vi "Generic command handler.vi"(8 "error in (no error)":errorcluster, 10 "Message in":refnum<class "GenericMessage.lvclass">, 11 "Tomo in":refnum<class "Tomo.lvclass">) -> (0 "error out":errorcluster, 2 "value":string, 3 "Tomo out":refnum<class "Tomo.lvclass">)   [LabVIEW 2012, in "Tomo.lvclass"]
doc: "The generic_command_handler processes the command 'generic'. Commands which are not part of the predefined list of commands fall under the 'generic' command for special activity."
uses:
  Tomo.lvclass
  <vilib>/Distrio/Murmex/GenericMessage/GenericMessage.lvclass
  <vilib>/Distrio/Murmex/Murmex/Murmex.lvclass
  <vilib>/Distrio/Murmex/StartMessage/StartMessage.lvclass
  file type.ctl
  notice type.ctl
  <vilib>/Distrio/Murmex/StopMessage/StopMessage.lvclass
  <vilib>/Distrio/Murmex/Message/Add or replace parameter.vi
  <vilib>/Distrio/Murmex/Message/Message.lvclass
panel:
  # "This method is called when the GENERIC\ntrigger is sent. \n\nOverride this method when your component needs to\nrespond to this trigger. \n\nCall parent for proper implementation"
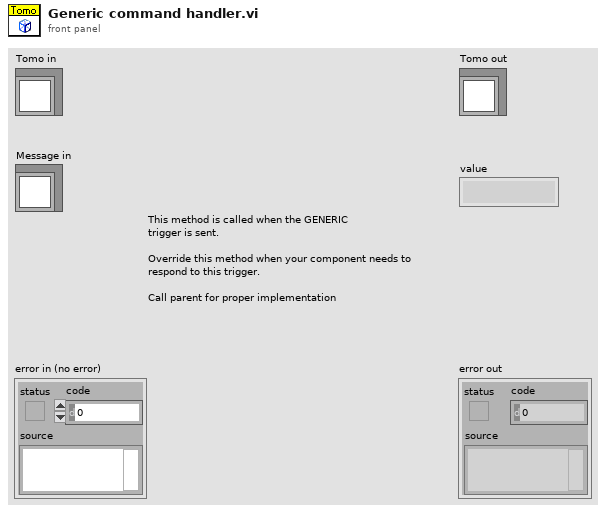
[diagram p1: front panel]
types:
  T1 = typedef "Tomo.lvclass/file type.ctl" = enum16{"Volume map", "Completed stacks"}
  T2 = typedef "Tomo.lvclass/notice type.ctl" = enum16{"Tomography stopped", "Tomography error", "Tomography finished", "Timing issue", "Critical timing issue"}
  T3 = typedef "Tomo.lvclass/volume map.ctl" = enum16{"Cubic volume", "Custom volume", "Self-generate volume"}
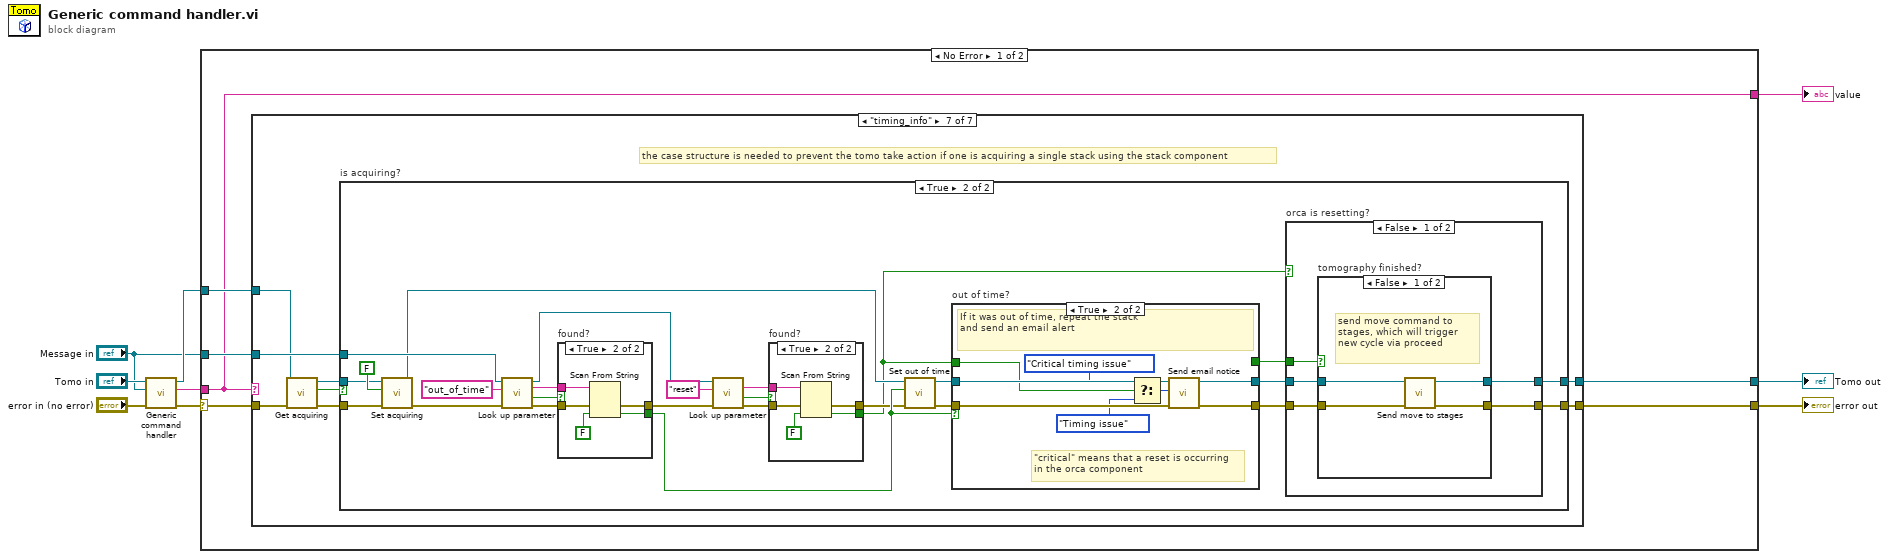
[diagram p0: block diagram]
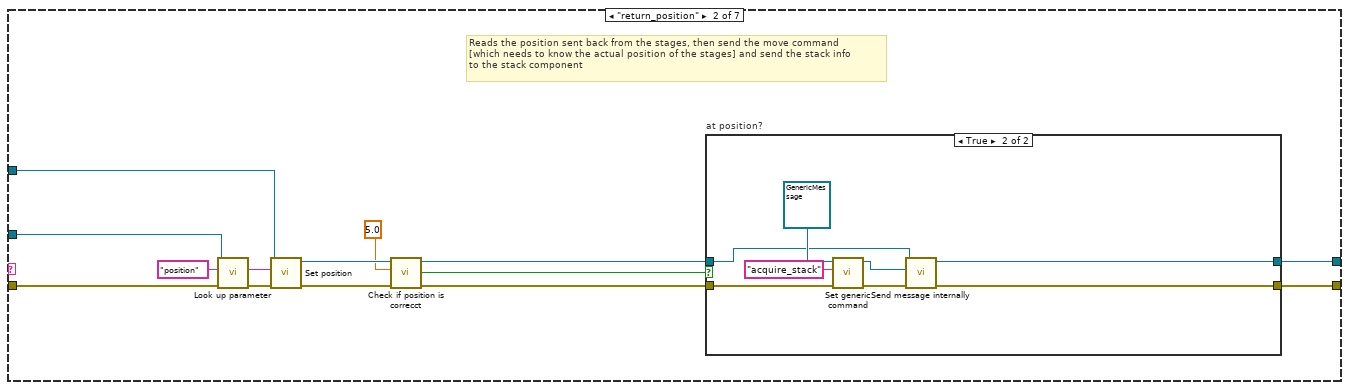
[diagram p3: hidden frame]
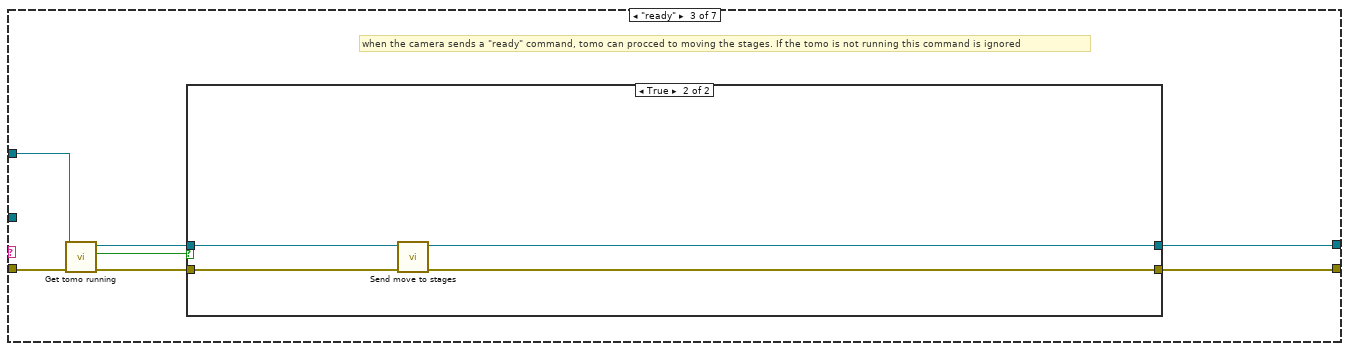
[diagram p5: hidden frame]
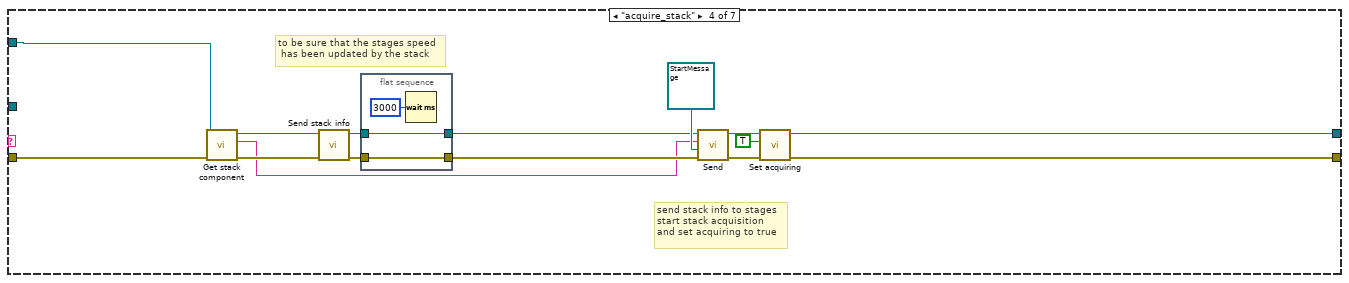
[diagram p7: hidden frame]
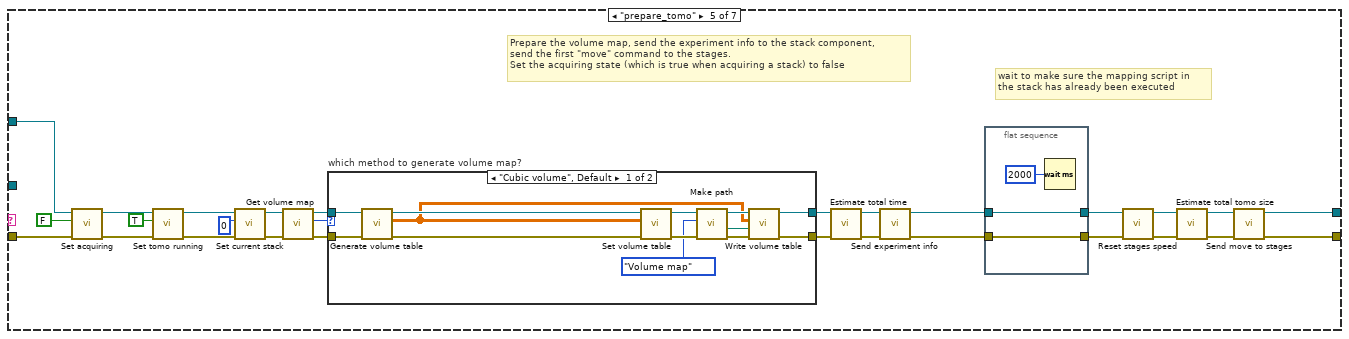
[diagram p8: hidden frame]
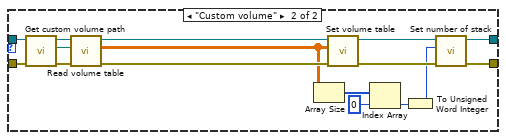
[diagram p9: hidden frame]
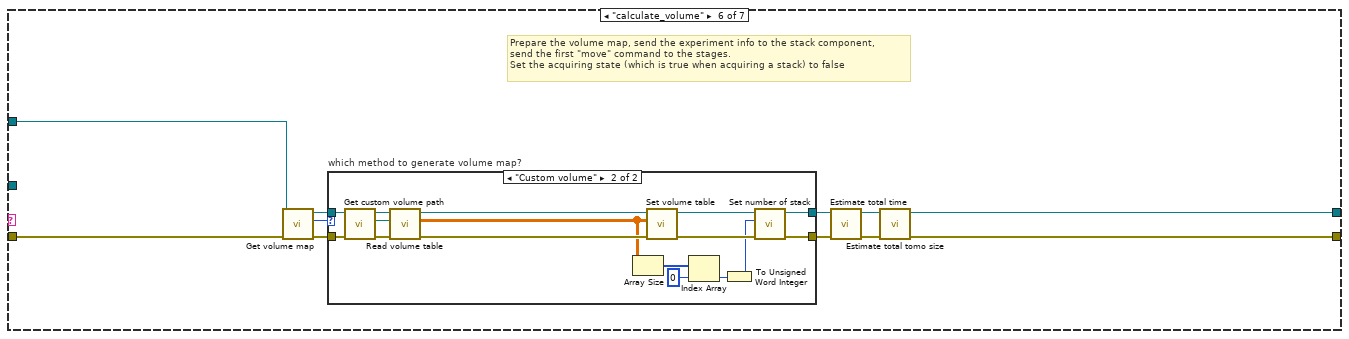
[diagram p10: hidden frame]
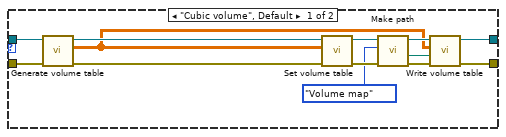
[diagram p11: hidden frame]
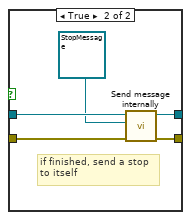
[diagram p13: hidden frame]
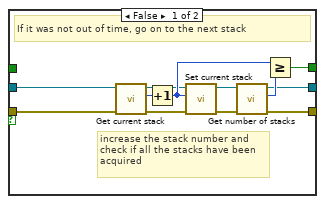
[diagram p16: hidden frame]
diagram:
  n1 = call-parent "Generic command handler.vi"("error in (no error)"="error in (no error)", "Message in"="Message in", "Murmex in"="Tomo in") -> ("error out"=w7:errorcluster, "value"=w6:string, "Murmex out"=w5:refnum<class "Tomo.lvclass">)  [unwired: 6 in]
  n2 = case shown="No Error" w7 {
    selector: w7 -> [w15 w257]
    tunnel: w6 -> [w11 w259]
    tunnel: w5 -> [w14 w258]
    tunnel: "Message in" -> [w13 _]
    tunnel: [w12 w258] -> w3
    tunnel: [w11 w259] -> w2
    tunnel: [w10 w257] -> w1
    frame No Error {
      n3 = case shown="\"timing_info\"" w11 {
        tunnel: w15 -> [w17 w31 w48 w61 w93 w139 w177]
        tunnel: w14 -> [w16 w30 w47 w59 w91 w138 w175]
        tunnel: w13 -> [_ w29 _ _ _ _ w180]
        tunnel: [w17 w19 w44 w56 w86 w135 w178] -> w10
        tunnel: [w16 w18 w42 w55 w85 w133 w179] -> w12
        frame Default {
        }
        frame "return_position" {
          # "Reads the position sent back from the stages, then send the move command\n[which needs to know the actual position of the stages] and send the stack info\nto the stack component"
          n4 = call <vilib>:"Look up parameter.vi"("error in (no error)"=w31, "name"="position", "Message in"=w29) -> ("error out"=w27:errorcluster, "key"=w26:string)  [unwired: 5 in, 2 out]
          n5 = call-dynamic "Set position.vi"("error in (no error)"=w27, "XML in"=w26, "Tomo in"=w30) -> ("error out"=w25:errorcluster, "Tomo out"=w24:refnum<class "Tomo.lvclass">)  [unwired: 7 in]
          n6 = call-dynamic "Check if position is correcct.vi"("error in (no error)"=w25, "Tolerance (um)"=5.0 ("Tolerance"), "Tomo in"=w24) -> ("error out"=w21:errorcluster, "correct?"=w22:bool, "Tomo out"=w20:refnum<class "Tomo.lvclass">)  [unwired: 6 in]
          n7 = case "at position?" shown="True" w22 {
            tunnel: w21 -> [w33 w40]
            tunnel: w20 -> [w32 w36]
            tunnel: [w33 w35] -> w19
            tunnel: [w32 w34] -> w18
            frame False {
            }
            frame True {
              n8 = call <vilib>:"Set generic command.vi"("error in (no error)"=w40, "generic command"="acquire_stack", "GenericMessage in"=refnum<class "GenericMessage.lvclass"> refnum ("Distrio Murmex 1.2:GenericMessage")) -> ("error out"=w41:errorcluster, "GenericMessage out"=w37:refnum<class "GenericMessage.lvclass">)  [unwired: 7 in]
              n9 = call <vilib>:"Send message internally.vi"("error in (no error)"=w41, "Message"=w37, "Murmex in"=w36) -> ("error out"=w35:errorcluster, "Murmex out"=w34:refnum<class "Tomo.lvclass">)  [unwired: 7 in]
            }
          }
        }
        frame "ready" {
          # "when the camera sends a \"ready\" command, tomo can procced to moving the stages. If the tomo is not running this command is ignored"
          n10 = call-dynamic "Get tomo running.vi"("error in (no error)"=w48, "Tomo in"=w47) -> ("error out"=w45:errorcluster, "tomo running?"=w46:bool, "Tomo out"=w43:refnum<class "Tomo.lvclass">)  [unwired: 7 in]
          n11 = case shown="True" w46 {
            tunnel: w45 -> [w49 w54]
            tunnel: [w49 w53] -> w44
            tunnel: w43 -> [w50 w52]
            tunnel: [w50 w51] -> w42
            frame False {
            }
            frame True {
              n12 = call-dynamic "Send move to stages.vi"("error in (no error)"=w54, "Tomo in"=w52) -> ("error out"=w53:errorcluster, "Tomo out"=w51:refnum<class "Tomo.lvclass">)  [unwired: 8 in]
            }
          }
        }
        frame "acquire_stack" {
          # "to be sure that the stages speed\n has been updated by the stack"
          # "send stack info to stages\nstart stack acquisition\nand set acquiring to true"
          n13 = call-dynamic "Get stack component.vi"("error in (no error)"=w61, "Tomo in"=w59) -> ("error out"=w60:errorcluster, "stack component"=w57:string, "Tomo out"=w58:refnum<class "Tomo.lvclass">)  [unwired: 7 in]
          n14 = call-dynamic "Send stack info.vi"("error in (no error)"=w60, "Tomo in"=w58) -> ("error out"=w62:errorcluster, "Tomo out"=w64:refnum<class "Tomo.lvclass">)  [unwired: 8 in]
          n15 = flat-sequence {
            tunnel: [w72] -> w65
            tunnel: w64 -> [w72]
            tunnel: [w71] -> w63
            tunnel: w62 -> [w71]
            frame #0 {
              n16 = Wait (ms)(milliseconds to wait=u32 3000) -> ()  [unwired: 1 out]
            }
          }
          n17 = call <vilib>:"Send.vi"("error in (no error)"=w63, "Message"=refnum<class "StartMessage.lvclass"> refnum ("Message in"), "recipient"=w57, "Murmex in"=w65) -> ("error out"=w69:errorcluster, "Murmex out"=w68:refnum<class "Tomo.lvclass">)  [unwired: 6 in]
          n18 = call-dynamic "Set acquiring.vi"("error in (no error)"=w69, "is acquiring?"=TRUE, "Tomo in"=w68) -> ("error out"=w56:errorcluster, "Tomo out"=w55:refnum<class "Tomo.lvclass">)  [unwired: 7 in]
        }
        frame "prepare_tomo" {
          # "wait to make sure the mapping script in \nthe stack has already been executed"
          # "Prepare the volume map, send the experiment info to the stack component,\nsend the first \"move\" command to the stages.\nSet the acquiring state (which is true when acquiring a stack) to false"
          n19 = call-dynamic "Set acquiring.vi"("error in (no error)"=w93, "is acquiring?"=FALSE, "Tomo in"=w91) -> ("error out"=w92:errorcluster, "Tomo out"=w82:refnum<class "Tomo.lvclass">)  [unwired: 7 in]
          n20 = call-dynamic "Set tomo running.vi"("error in (no error)"=w92, "tomo running?"=TRUE, "Tomo in"=w82) -> ("error out"=w77:errorcluster, "Tomo out"=w78:refnum<class "Tomo.lvclass">)  [unwired: 7 in]
          n21 = call-dynamic "Set current stack.vi"("error in (no error)"=w77, "Current stack"=u16 0, "Tomo in"=w78) -> ("error out"=w96:errorcluster, "Tomo out"=w97:refnum<class "Tomo.lvclass">)  [unwired: 7 in]
          n22 = call-dynamic "Get volume map.vi"("error in (no error)"=w96, "Tomo in"=w97) -> ("error out"=w99:errorcluster, "Volume map"=w100:T3, "Tomo out"=w98:refnum<class "Tomo.lvclass">)  [unwired: 7 in]
          n23 = case "which method to generate volume map?" shown="\"Cubic volume\", Default" w100 {
            tunnel: w99 -> [w115 w130]
            tunnel: w98 -> [w116 w128]
            tunnel: [w105 w122] -> w88
            tunnel: [w104 w124] -> w94
            frame "Cubic volume", Default {
              n24 = call-dynamic "Generate volume table.vi"("error in (no error)"=w115, "Tomo in"=w116) -> ("error out"=w113:errorcluster, "Volume table"=w106:dbl[][], "Tomo out"=w114:refnum<class "Tomo.lvclass">)  [unwired: 7 in]
              n25 = call-dynamic "Set volume table.vi"("error in (no error)"=w113, "Volume map in"=w106, "Tomo in"=w114) -> ("error out"=w111:errorcluster, "Tomo out"=w112:refnum<class "Tomo.lvclass">)  [unwired: 7 in]
              n26 = call-dynamic "Make path.vi"("error in (no error)"=w111, "File type"=file_type."Volume map", "Tomo in"=w112) -> ("error out"=w108:errorcluster, "path"=w107:path, "Tomo out"=w109:refnum<class "Tomo.lvclass">)  [unwired: 6 in]
              n27 = call-dynamic "Write volume table.vi"("error in (no error)"=w108, "File name"=w107, "Volume map"=w106, "Tomo in"=w109) -> ("error out"=w104:errorcluster, "Tomo out"=w105:refnum<class "Tomo.lvclass">)  [unwired: 6 in]
            }
            frame "Custom volume" {
              n28 = call-dynamic "Get custom volume path.vi"("error in (no error)"=w130, "Tomo in"=w128) -> ("error out"=w129:errorcluster, "Custom volume path"=w126:path, "Tomo out"=w127:refnum<class "Tomo.lvclass">)  [unwired: 7 in]
              n29 = call-dynamic "Read volume table.vi"("error in (no error)"=w129, "File path"=w126, "Tomo in"=w127) -> ("error out"=w131:errorcluster, "System Array"=w118:dbl[][], "Tomo out"=w132:refnum<class "Tomo.lvclass">)  [unwired: 6 in]
              n30 = Array Size(array=w118) -> (size(s)=w121:i32[])
              n31 = call-dynamic "Set volume table.vi"("error in (no error)"=w131, "Volume map in"=w118, "Tomo in"=w132) -> ("error out"=w125:errorcluster, "Tomo out"=w123:refnum<class "Tomo.lvclass">)  [unwired: 7 in]
              n32 = Index Array(array=w121, index=0) -> (element=w119:i32)
              n33 = To Unsigned Word Integer(number=w119) -> (unsigned 16bit integer=w117:u16)
              n34 = call-dynamic "Set number of stack.vi"("error in (no error)"=w125, "Number of stacks"=w117, "Tomo in"=w123) -> ("error out"=w124:errorcluster, "Tomo out"=w122:refnum<class "Tomo.lvclass">)  [unwired: 7 in]
            }
          }
          n35 = call-dynamic "Estimate total time.vi"("error in (no error)"=w94, "Tomo in"=w88) -> ("error out"=w89:errorcluster, "Tomo out"=w87:refnum<class "Tomo.lvclass">)  [unwired: 8 in]
          n36 = call-dynamic "Send experiment info.vi"("error in (no error)"=w89, "Tomo in"=w87) -> ("error out"=w73:errorcluster, "Tomo out"=w75:refnum<class "Tomo.lvclass">)  [unwired: 8 in]
          n37 = flat-sequence {
            tunnel: [w103] -> w76
            tunnel: w75 -> [w103]
            tunnel: [w102] -> w74
            tunnel: w73 -> [w102]
            frame #0 {
              n38 = Wait (ms)(milliseconds to wait=u32 2000) -> ()  [unwired: 1 out]
            }
          }
          n39 = call-dynamic "Reset stages speed.vi"("error in (no error)"=w74, "Tomo in"=w76) -> ("error out"=w80:errorcluster, "Tomo out"=w79:refnum<class "Tomo.lvclass">)  [unwired: 8 in]
          n40 = call "Estimate total tomo size.vi"("error in (no error)"=w80, "Tomo in"=w79) -> ("error out"=w84:errorcluster, "Tomo out"=w83:refnum<class "Tomo.lvclass">)  [unwired: 7 in, 1 out]
          n41 = call-dynamic "Send move to stages.vi"("error in (no error)"=w84, "Tomo in"=w83) -> ("error out"=w86:errorcluster, "Tomo out"=w85:refnum<class "Tomo.lvclass">)  [unwired: 8 in]
        }
        frame "calculate_volume" {
          # "Prepare the volume map, send the experiment info to the stack component,\nsend the first \"move\" command to the stages.\nSet the acquiring state (which is true when acquiring a stack) to false"
          n42 = call-dynamic "Get volume map.vi"("error in (no error)"=w139, "Tomo in"=w138) -> ("error out"=w142:errorcluster, "Volume map"=w143:T3, "Tomo out"=w141:refnum<class "Tomo.lvclass">)  [unwired: 7 in]
          n43 = case "which method to generate volume map?" shown="\"Custom volume\"" w143 {
            tunnel: w142 -> [w155 w170]
            tunnel: w141 -> [w156 w168]
            tunnel: [w145 w162] -> w137
            tunnel: [w144 w164] -> w140
            frame "Cubic volume", Default {
              n44 = call-dynamic "Generate volume table.vi"("error in (no error)"=w155, "Tomo in"=w156) -> ("error out"=w153:errorcluster, "Volume table"=w146:dbl[][], "Tomo out"=w154:refnum<class "Tomo.lvclass">)  [unwired: 7 in]
              n45 = call-dynamic "Set volume table.vi"("error in (no error)"=w153, "Volume map in"=w146, "Tomo in"=w154) -> ("error out"=w151:errorcluster, "Tomo out"=w152:refnum<class "Tomo.lvclass">)  [unwired: 7 in]
              n46 = call-dynamic "Make path.vi"("error in (no error)"=w151, "File type"=file_type."Volume map", "Tomo in"=w152) -> ("error out"=w148:errorcluster, "path"=w147:path, "Tomo out"=w149:refnum<class "Tomo.lvclass">)  [unwired: 6 in]
              n47 = call-dynamic "Write volume table.vi"("error in (no error)"=w148, "File name"=w147, "Volume map"=w146, "Tomo in"=w149) -> ("error out"=w144:errorcluster, "Tomo out"=w145:refnum<class "Tomo.lvclass">)  [unwired: 6 in]
            }
            frame "Custom volume" {
              n48 = call-dynamic "Get custom volume path.vi"("error in (no error)"=w170, "Tomo in"=w168) -> ("error out"=w169:errorcluster, "Custom volume path"=w166:path, "Tomo out"=w167:refnum<class "Tomo.lvclass">)  [unwired: 7 in]
              n49 = call-dynamic "Read volume table.vi"("error in (no error)"=w169, "File path"=w166, "Tomo in"=w167) -> ("error out"=w171:errorcluster, "System Array"=w158:dbl[][], "Tomo out"=w172:refnum<class "Tomo.lvclass">)  [unwired: 6 in]
              n50 = Array Size(array=w158) -> (size(s)=w161:i32[])
              n51 = call-dynamic "Set volume table.vi"("error in (no error)"=w171, "Volume map in"=w158, "Tomo in"=w172) -> ("error out"=w165:errorcluster, "Tomo out"=w163:refnum<class "Tomo.lvclass">)  [unwired: 7 in]
              n52 = Index Array(array=w161, index=0) -> (element=w159:i32)
              n53 = To Unsigned Word Integer(number=w159) -> (unsigned 16bit integer=w157:u16)
              n54 = call-dynamic "Set number of stack.vi"("error in (no error)"=w165, "Number of stacks"=w157, "Tomo in"=w163) -> ("error out"=w164:errorcluster, "Tomo out"=w162:refnum<class "Tomo.lvclass">)  [unwired: 7 in]
            }
          }
          n55 = call-dynamic "Estimate total time.vi"("error in (no error)"=w140, "Tomo in"=w137) -> ("error out"=w136:errorcluster, "Tomo out"=w134:refnum<class "Tomo.lvclass">)  [unwired: 8 in]
          n56 = call "Estimate total tomo size.vi"("error in (no error)"=w136, "Tomo in"=w134) -> ("error out"=w135:errorcluster, "Tomo out"=w133:refnum<class "Tomo.lvclass">)  [unwired: 7 in, 1 out]
        }
        frame "timing_info" {
          # "the case structure is needed to prevent the tomo take action if one is acquiring a single stack using the stack component"
          n57 = call-dynamic "Get acquiring.vi"("error in (no error)"=w177, "Tomo in"=w175) -> ("error out"=w176:errorcluster, "is acquiring?"=w173:bool, "Tomo out"=w174:refnum<class "Tomo.lvclass">)  [unwired: 7 in]
          n58 = case "is acquiring?" shown="True" w173 {
            tunnel: w180 -> [_ w208]
            tunnel: [w182 w201] -> w179
            tunnel: [w181 w200] -> w178
            tunnel: w176 -> [w181 w197]
            tunnel: w174 -> [w182 w195]
            frame False {
            }
            frame True {
              n59 = call-dynamic "Set acquiring.vi"("error in (no error)"=w197, "is acquiring?"=FALSE, "Tomo in"=w195) -> ("error out"=w196:errorcluster, "Tomo out"=w193:refnum<class "Tomo.lvclass">)  [unwired: 7 in]
              n60 = call <vilib>:"Look up parameter.vi"("error in (no error)"=w196, "name"="out_of_time", "Message in"=w208) -> ("error out"=w206:errorcluster, "found?"=w204:bool, "key"=w205:string, "Message out"=w185:refnum<class "GenericMessage.lvclass">)  [unwired: 5 in]
              n61 = case "found?" shown="True" w204 {
                tunnel: w206 -> [w251 w255]
                tunnel: w205 -> [_ w254]
                tunnel: [w251 w253] -> w184
                tunnel: [_ w252] -> w191
                frame False {
                }
                frame True {
                  n62 = Scan From String(input string=w254, error in=w255, default 1=FALSE) -> (error out=w253:errorcluster, output 1=w252:bool)  [unwired: 2 in, 2 out]
                }
              }
              n63 = call <vilib>:"Look up parameter.vi"("error in (no error)"=w184, "name"="reset", "Message in"=w185) -> ("error out"=w189:errorcluster, "found?"=w187:bool, "key"=w188:string)  [unwired: 5 in, 1 out]
              n64 = case "found?" shown="True" w187 {
                tunnel: w189 -> [w225 w229]
                tunnel: w188 -> [_ w228]
                tunnel: [w225 w227] -> w186
                tunnel: [_ w226] -> w183
                frame False {
                }
                frame True {
                  n65 = Scan From String(input string=w228, error in=w229, default 1=FALSE) -> (error out=w227:errorcluster, output 1=w226:bool)  [unwired: 2 in, 2 out]
                }
              }
              n66 = call-dynamic "Set out of time.vi"("error in (no error)"=w186, "out of time?"=w191, "Tomo in"=w193) -> ("error out"=w194:errorcluster, "Tomo out"=w192:refnum<class "Tomo.lvclass">)  [unwired: 7 in]
              n67 = case "out of time?" shown="True" w191 {
                tunnel: w194 -> [w235 w249]
                tunnel: w192 -> [w234 w250]
                tunnel: [w233 w248] -> w203
                tunnel: [w232 w247] -> w202
                tunnel: [w231 _] -> w199
                tunnel: w183 -> [_ w244]
                frame False {
                  # "increase the stack number and\ncheck if all the stacks have been\nacquired"
                  # "If it was not out of time, go on to the next stack"
                  n68 = call-dynamic "Get current stack.vi"("error in (no error)"=w235, "Tomo in"=w234) -> ("error out"=w237:errorcluster, "Current stack"=w238:u16, "Tomo out"=w236:refnum<class "Tomo.lvclass">)  [unwired: 7 in]
                  n69 = Increment(x=w238) -> (x+1=w242:u16)
                  n70 = call-dynamic "Set current stack.vi"("error in (no error)"=w237, "Current stack"=w242, "Tomo in"=w236) -> ("error out"=w239:errorcluster, "Tomo out"=w240:refnum<class "Tomo.lvclass">)  [unwired: 7 in]
                  n71 = call-dynamic "Get number of stacks.vi"("error in (no error)"=w239, "Tomo in"=w240) -> ("error out"=w233:errorcluster, "Number of stacks"=w241:u16, "Tomo out"=w232:refnum<class "Tomo.lvclass">)  [unwired: 7 in]
                  n72 = Greater Or Equal?(x=w242, y=w241) -> (x >= y?=w231:bool)
                }
                frame True {
                  # "\"critical\" means that a reset is occurring\nin the orca component"
                  # "If it was out of time, repeat the stack\nand send an email alert"
                  n73 = Select(t=notice_type."Critical timing issue" ("Notice type"), s=w244, f=notice_type."Timing issue" ("Notice type")) -> (s? t:f=w243:T2)
                  n74 = call-dynamic "Send email notice.vi"("error in (no error)"=w249, "Notice type"=w243, "Tomo in"=w250) -> ("error out"=w248:errorcluster, "Tomo out"=w247:refnum<class "Tomo.lvclass">)  [unwired: 7 in]
                }
              }
              n75 = case "orca is resetting?" shown="False" w183 {
                tunnel: w203 -> [w213 w224]
                tunnel: w202 -> [w212 w223]
                tunnel: [w211 w223] -> w201
                tunnel: [w210 w224] -> w200
                tunnel: w199 -> [w209 _]
                frame False {
                  n76 = case "tomography finished?" shown="False" w209 {
                    tunnel: w213 -> [w217 w222]
                    tunnel: w212 -> [w216 w219]
                    tunnel: [w215 w220] -> w211
                    tunnel: [w214 w221] -> w210
                    frame False {
                      # "send move command to stages, which will trigger new cycle via proceed"
                      n77 = call-dynamic "Send move to stages.vi"("error in (no error)"=w217, "Tomo in"=w216) -> ("error out"=w214:errorcluster, "Tomo out"=w215:refnum<class "Tomo.lvclass">)  [unwired: 8 in]
                    }
                    frame True {
                      # "if finished, send a stop\nto itself"
                      n78 = call <vilib>:"Send message internally.vi"("error in (no error)"=w222, "Message"=refnum<class "StopMessage.lvclass"> refnum ("Message in"), "Murmex in"=w219) -> ("error out"=w221:errorcluster, "Murmex out"=w220:refnum<class "Tomo.lvclass">)  [unwired: 7 in]
                    }
                  }
                }
                frame True {
                  # "do nothing. Orca will tell\nyou when it's ready"
                }
              }
            }
          }
        }
      }
    }
    frame Error {
    }
  }
  "error out" <- w1
  "Tomo out" <- w3
  "value" <- w2
